vi "add line to table.vi"(8 "error in":errorcluster, 10 "line":T1, 11 "operations table":T2) -> (0 "error out":errorcluster)   [LabVIEW 2013, in "CVT editor node.lvclass"]
uses:
  CVT editor node.lvclass
  table reference.ctl
  table line.ctl
  <vilib>/NI/Tag Bus Module Framework/channel/TBM channel.lvclass
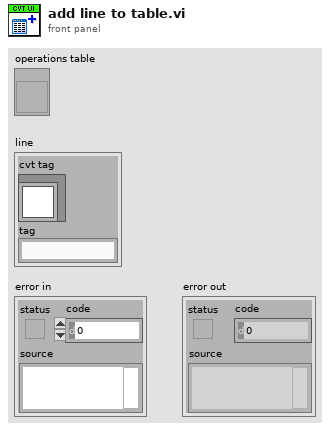
[diagram p1: front panel]
types:
  T1 = typedef "CVT editor node.lvclass/table line.ctl" = cluster{"cvt tag":refnum<class "TBM channel.lvclass">, "tag":string}
  T2 = typedef "CVT editor node.lvclass/table reference.ctl" = refnum<vi>
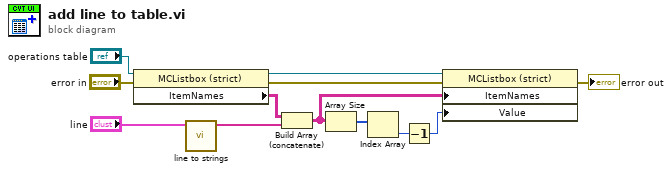
[diagram p0: block diagram]
diagram:
  n1 = property class="MCListbox (strict)"(reference="operations table", error in="error in") -> (reference out=w6:T2, error out=w7:errorcluster, "ItemNames"=w8:string[][])
  n2 = call "line to strings.vi"("line"="line") -> ("strings"=w9:string[])  [unwired: 10 in]
  n3 = Build Array (concatenate)(w8, w9) -> (w5:string[][])
  n4 = Array Size(array=w5) -> (size(s)=w4:i32[])
  n5 = Index Array(array=w4) -> (element=w3:i32)  [unwired: 1 in]
  n6 = Decrement(x=w3) -> (x-1=w1:i32)
  n7 = property class="MCListbox (strict)"(reference=w6, error in=w7, "ItemNames"=w5, "Value"=w1) -> (error out=→"error out":errorcluster)  [unwired: 1 out]
